vi "Auto 4.vi"(8 "Error In":errorcluster) -> (0 "Error Out":errorcluster)   [LabVIEW 2014]
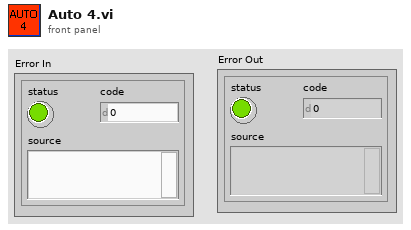
[diagram p1: front panel]
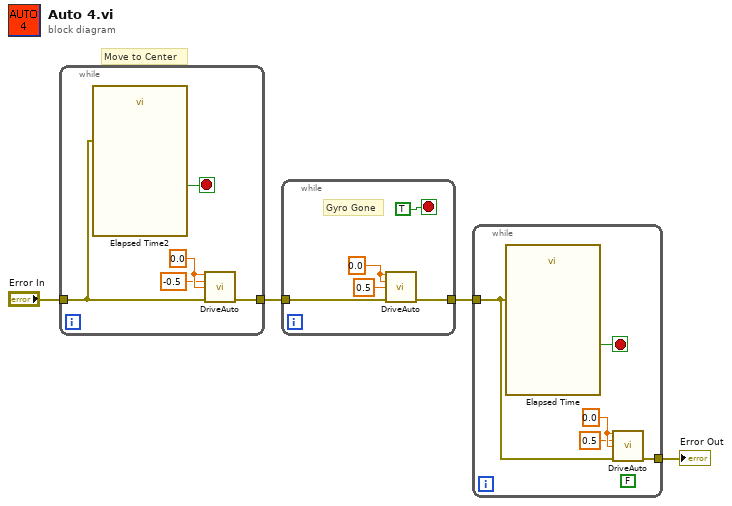
[diagram p0: block diagram]
diagram:
  # "Move to Center"
  n1 = while {
    tunnel: "Error In" -> [w5]
    tunnel: [w9] -> w3
    stop <- w6 stop-if-true
    w8 = 0.0 ("Arm Value")
    n2 = call "Elapsed Time2"("error in (no error)"=w5) -> ("Time has Elapsed"=w6:bool)  [unwired: 11 in, 7 out]
    n3 = call "DriveAuto.vi"("X In"=w8, "Y In"=-0.5 ("X In"), "R In"=w8, "Error In"=w5) -> ("Error Out"=w9:errorcluster)  [unwired: 11 in]
  }
  n4 = while {
    tunnel: w3 -> [w14]
    tunnel: [w13] -> w4
    stop <- TRUE stop-if-true
    w12 = 0.0 ("Arm Value")
    # "Gyro Gone"
    n5 = call "DriveAuto.vi"("X In"=w12, "Y In"=w12, "R In"=0.5 ("X In"), "Error In"=w14) -> ("Error Out"=w13:errorcluster)  [unwired: 11 in]
  }
  n6 = while {
    tunnel: w4 -> [w15]
    tunnel: [w19] -> w1
    stop <- w16 stop-if-true
    (unwired) FALSE ("Grabber Open/Close")
    w18 = 0.0 ("Arm Value")
    n7 = call "Elapsed Time"("error in (no error)"=w15) -> ("Time has Elapsed"=w16:bool)  [unwired: 11 in, 7 out]
    n8 = call "DriveAuto.vi"("X In"=w18, "Y In"=0.5 ("X In"), "R In"=w18, "Error In"=w15) -> ("Error Out"=w19:errorcluster)  [unwired: 11 in]
  }
  "Error Out" <- w1
